vi "1 DIMENSION AND 2 DIMENSIONAL ARRAY.vi"() -> ()   [LabVIEW 2019]
panel:
  in  "4-DIMENSIONAL ARRAY":dbl[][][][](array[numeric])=[[[[10.0, 20.0, 30.0, 40.0], [50.0, 60.0, 70.0, 80.0], [90.0, 100.0, 110.0, 120.0], [130.0, 140.0, 150.0, 160.0], [170.0, 180.0, 190.0, 200.0]]]]
  out "4-DIMENSIONAL ARRAY 2":dbl[][][][](array[numeric])
  out "3-DIMENSIONAL ARRAY 2":dbl[][][](array[numeric])
  out "2-DIMENSIONAL ARRAY 2":dbl[][](array[numeric])
  out "1-DIMENSION ARRAY 2":dbl[](array[numeric])
  out "Numeric 2":dbl
  in  "3-DIMENSIONAL ARRAY":dbl[][][](array[numeric])=[[[10.0, 20.0, 30.0, 40.0], [50.0, 60.0, 70.0, 80.0], [90.0, 100.0, 110.0, 120.0], [130.0, 140.0, 150.0, 160.0], [170.0, 180.0, 190.0, 200.0]]]
  in  "2-DIMENSIONAL ARRAY":dbl[][](array[numeric])=[[10.0, 20.0, 30.0], [40.0, 50.0, 60.0], [70.0, 80.0, 90.0], [100.0, 110.0, 120.0], [130.0, 140.0, 150.0]]
  in  "Numeric":dbl=10.0
  in  "1-DIMENSION ARRAY":dbl[](array[numeric])=[10.0, 20.0, 30.0, 40.0, 50.0]
  # "SINGLE AND MULTI-DIMENSIONAL ARRAY"
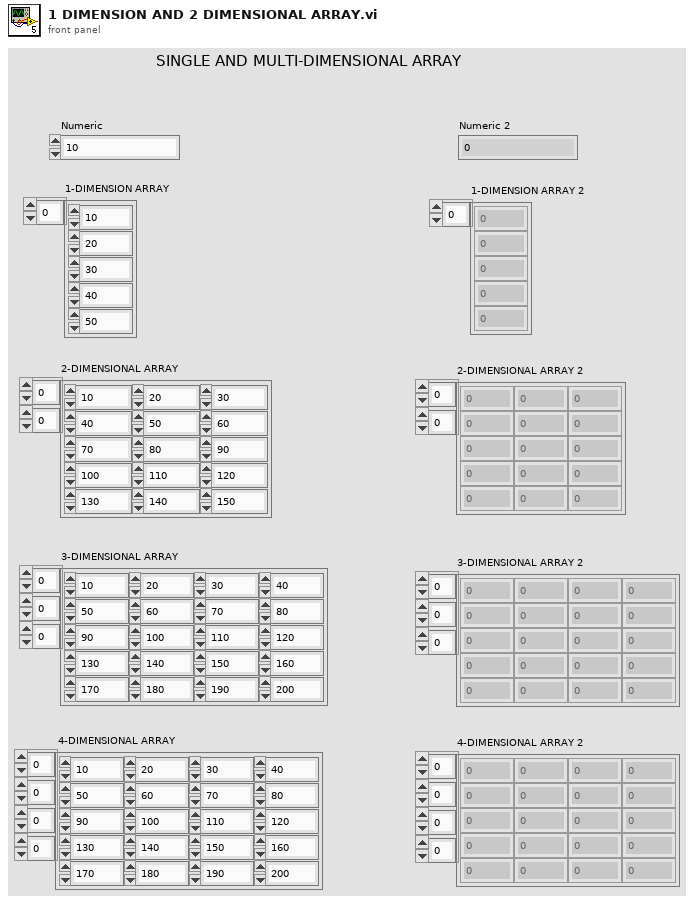
[diagram p1: front panel]
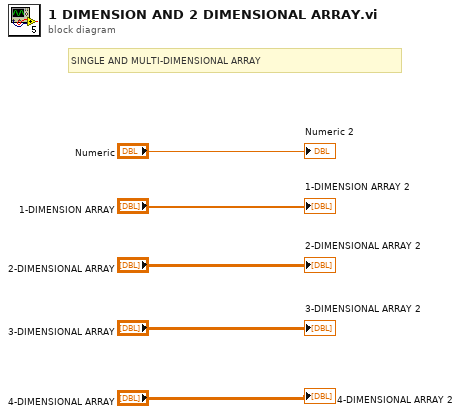
[diagram p0: block diagram]
diagram:
  # "SINGLE AND MULTI-DIMENSIONAL ARRAY"
  "Numeric 2" <- "Numeric"
  "1-DIMENSION ARRAY 2" <- "1-DIMENSION ARRAY"
  "2-DIMENSIONAL ARRAY 2" <- "2-DIMENSIONAL ARRAY"
  "3-DIMENSIONAL ARRAY 2" <- "3-DIMENSIONAL ARRAY"
  "4-DIMENSIONAL ARRAY 2" <- "4-DIMENSIONAL ARRAY"
